vi "SalvaImpostazioni_OUTPUT.vi"(11 "Array Misure Output":dbl[](array[numeric])) -> ()   [LabVIEW 2016]
uses:
  TypeDef/ClusterCaratteristicheMisura_OUTPUT.ctl
panel:
  in  "Cluster Caratteriestiche Misura":T1
  in  "Array ClusterCaratteristicheMisura":T1[](array[typedef])
  in  "Salva Impostazioni":bool
  out "Numero di misure":i32
  in  "Carica Impostazioni":bool
  in  "Stop":bool
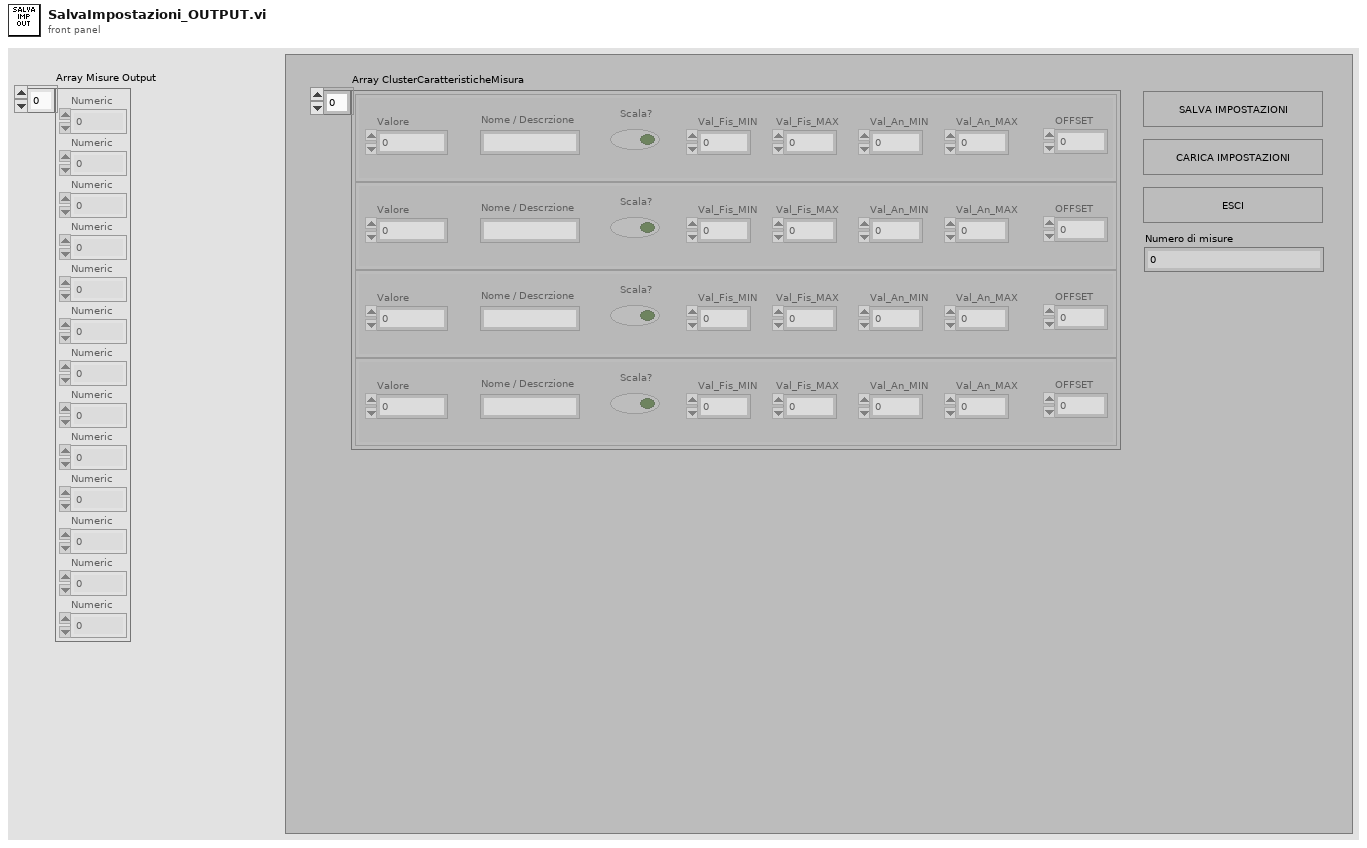
[diagram p1: front panel]
types:
  T1 = typedef "ClusterCaratteristicheMisura_OUTPUT.ctl" = cluster{"Nome / Descrzione":string, "Scala?":bool, "Val_Fis_MIN":dbl, "Val_Fis_MAX":dbl, "Val_An_MIN":dbl, "Val_An_MAX":dbl, "OFFSET":dbl, "Valore":dbl}
  T2 = typedef "ClusterCaratteristicheMisura_INPUT.ctl" = cluster{"Nome / Descrzione":string, "Scala?":bool, "Ai_MIN":dbl, "Ai_MAX":dbl, "RANGE":dbl, "OFFSET":dbl, "Unità di Misura":T3, "Valore":dbl}
  T3 = typedef "UnitàMisura.ctl" = enum16{"V", "mA", "Bar", "RPM", "m3/s", "m3/min", "m3/h", "l/s", "l/min", "in3/min", "ft3/min", "gpm", "igpm", "igph"}
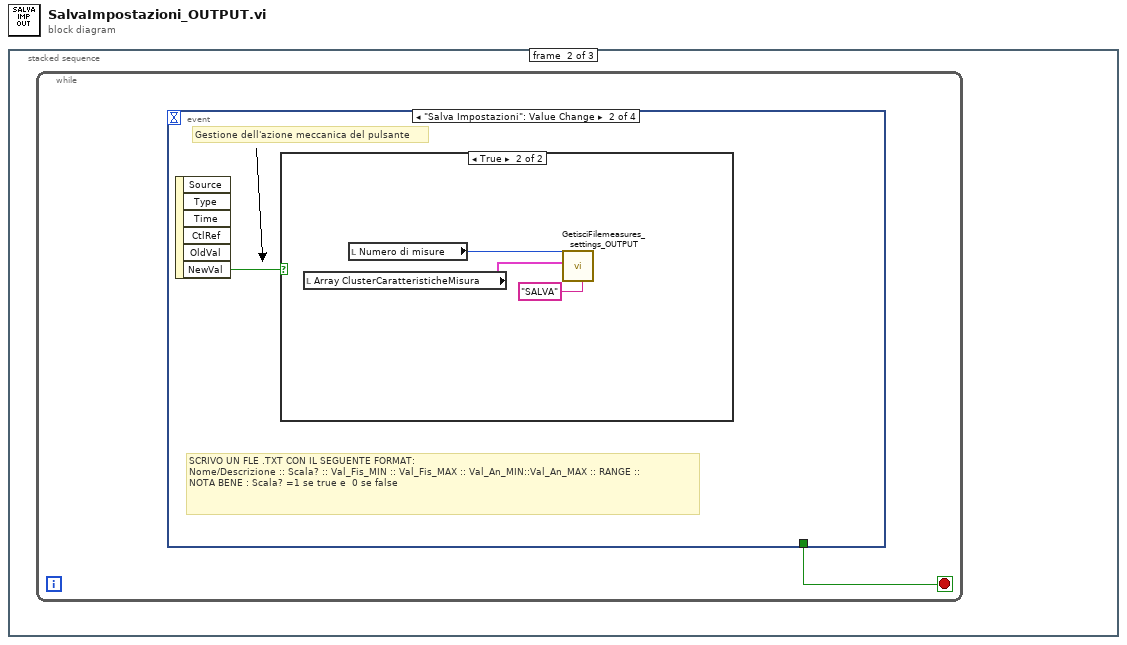
[diagram p0: block diagram]
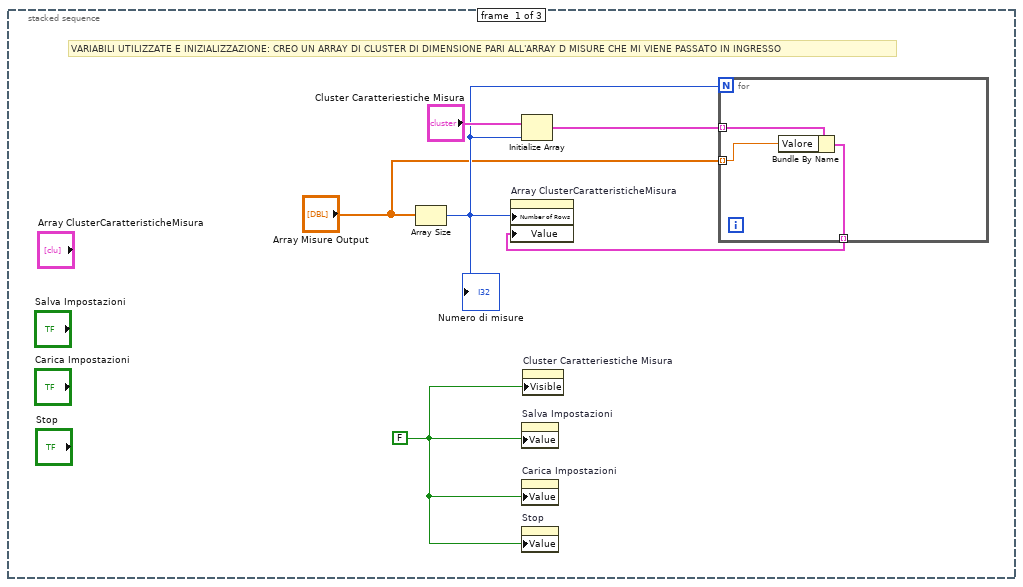
[diagram p2: hidden frame]
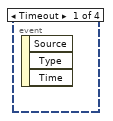
[diagram p3: hidden frame]
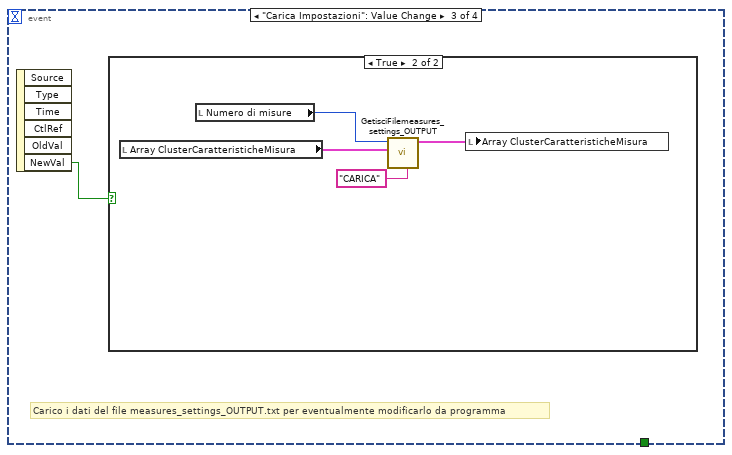
[diagram p5: hidden frame]
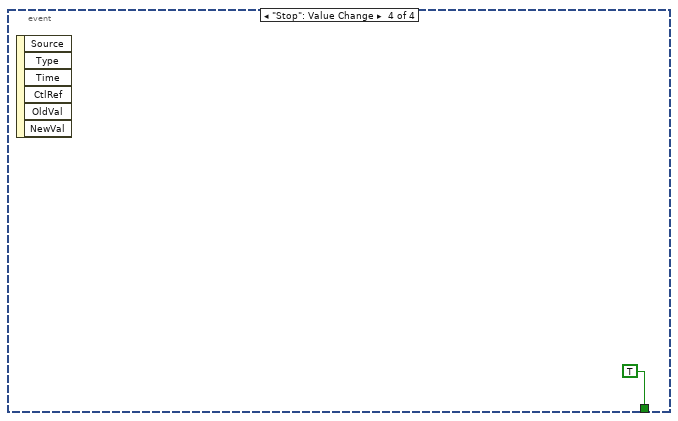
[diagram p7: hidden frame]
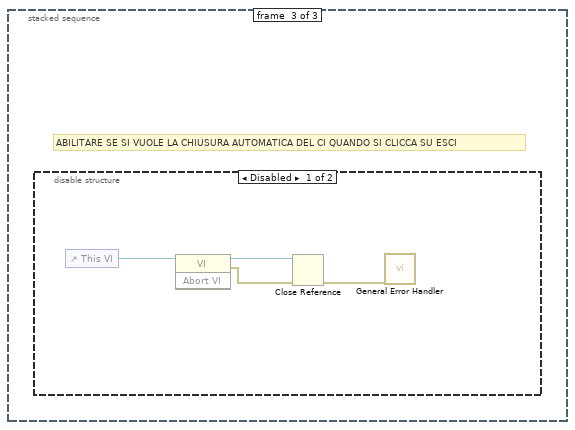
[diagram p8: hidden frame]
diagram:
  n1 = stacked-sequence {
    frame #0 {
      w6 = FALSE ("Salva Impostazioni")
      # "VARIABILI UTILIZZATE E INIZIALIZZAZIONE: CREO UN ARRAY DI CLUSTER DI DIMENSIONE PARI ALL'ARRAY D MISURE CHE MI VIENE PASSATO IN INGRESSO"
      n2 = Array Size(array="Array Misure Output") -> (size(s)=w3:i32)
      "Numero di misure" <- w3
      n3 = Initialize Array("Cluster Caratteriestiche Misura", w3) -> (w4:T1[])
      n4 = property on="Salva Impostazioni" class="Bool (strict)"("Value"=w6) -> ()  [unwired: 2 in, 2 out]
      n5 = property on="Carica Impostazioni" class="Bool (strict)"("Value"=w6) -> ()  [unwired: 2 in, 2 out]
      n6 = property on="Stop" class="Bool (strict)"("Value"=w6) -> ()  [unwired: 2 in, 2 out]
      n7 = property on="Cluster Caratteriestiche Misura" class="Clust (strict)"("Visible"=w6) -> ()  [unwired: 2 in, 2 out]
      n8 = for {
        N: w3 -> [_]
        tunnel: w4 -> [w9] mode=indexing
        tunnel: "Array Misure Output" -> [w8] mode=indexing
        tunnel: [w7] -> w1 mode=indexing
        n9 = Bundle By Name(cluster=w9, "Valore"=w8) -> (w7:T1)
      }
      n10 = property on="Array ClusterCaratteristicheMisura" class="Arr (strict)"("Number of Rows"=w3, "Value"=w1) -> ()  [unwired: 2 in, 2 out]
    }
    frame #1 {
      n11 = while {
        stop <- w10 stop-if-true
        n12 = event shown="[1] \"Salva Impostazioni\": Value Change" {
          selector: _ -> [_ _ _ _]
          dyn-events: _ -> [_ _ _ _]
          timeout: _ -> [_ _ _ _]
          tunnel: [_ _ _ TRUE] -> w10
          event Timeout {
            n13 = event-data() -> ()  [unwired: 1 in, 3 out]
          }
          event "Salva Impostazioni": Value Change {
            # "Gestione dell'azione meccanica del pulsante"
            # "SCRIVO UN FLE .TXT CON IL SEGUENTE FORMAT:\nNome/Descrizione :: Scala? :: Val_Fis_MIN :: Val_Fis_MAX :: Val_An_MIN::Val_An_MAX :: RANGE ::  \nNOTA BENE : Scala? =1 se true e  0 se false"
            n14 = event-data() -> ("NewVal"=w11:bool)  [unwired: 1 in, 5 out]
            n15 = case shown="True" w11 {
              frame False {
              }
              frame True {
                n16 = local read "Array ClusterCaratteristicheMisura"() -> (w13:T1[])
                n17 = local read "Numero di misure"() -> (w14:i32)
                n18 = call "GetisciFilemeasures_settings_OUTPUT.vi"("Azione"="SALVA", "Array ClusterCaratteristicheMisura IN"=w13, "Numero Misure"=w14) -> ()  [unwired: 8 in, 1 out]
              }
            }
          }
          event "Carica Impostazioni": Value Change {
            # "Carico i dati del file measures_settings_OUTPUT.txt per eventualmente modificarlo da programma"
            n19 = event-data() -> ("NewVal"=w15:bool)  [unwired: 1 in, 5 out]
            n20 = case shown="True" w15 {
              frame False {
              }
              frame True {
                n21 = local read "Array ClusterCaratteristicheMisura"() -> (w18:T1[])
                n22 = local read "Numero di misure"() -> (w17:i32)
                n23 = call "GetisciFilemeasures_settings_OUTPUT.vi"("Azione"="CARICA", "Array ClusterCaratteristicheMisura IN"=w18, "Numero Misure"=w17) -> ("Array ClusterCaratteristicheMisura OUT"=w16:T2[])  [unwired: 8 in]
                n24 = local write "Array ClusterCaratteristicheMisura"(w16) -> ()
              }
            }
          }
          event "Stop": Value Change {
            n25 = event-data() -> ()  [unwired: 1 in, 6 out]
          }
        }
      }
    }
    frame #2 {
      # "ABILITARE SE SI VUOLE LA CHIUSURA AUTOMATICA DEL CI QUANDO SI CLICCA SU ESCI"
      n26 = disable-structure shown="Disabled" {
        frame Disabled {
          n27 = control-ref of="This VI"() -> (w24:refnum<vi>)
          n28 = invoke class="VI" method="Abort VI"(reference=w24) -> (reference out=w23:refnum<vi>, error out=w21:errorcluster)  [unwired: 2 in, 1 out]
          n29 = Close Reference(reference=w23, error in (no error)=w21) -> (error out=w22:errorcluster)
          n30 = call <vilib>:"General Error Handler.vi"("error in (no error)"=w22) -> ()  [unwired: 10 in, 5 out]
        }
        frame Enabled {
        }
      }
    }
  }
